vi "test Ntrip-Client.vi"() -> ()   [LabVIEW 2019]
uses:
  <vilib>/Instr/_visa.llb/VISA Configure Serial Port (Instr).vi
panel:
  in  "탭 컨트롤":enum32{"Main", "ref"}(tab)
  out "RTCM recv":string
  in  "address":string="gnss.eseoul.go.kr"
  in  "remote port":u16=2101
  in  "bytes to read":i32=100000
  in  "stop":bool
  in  "VISA resource name":refnum<visa-resource-name> caption="GNSS port"
  in  "정지":bool
  in  "baud rate (9600)":u32=9600 caption="rate"
  in  "불리언":bool
  in  "데이터 입력":string
  # "GET /YONS-RTCM32-M5 HTTP/1.0\nUser-Agent: NTRIP YbbaekRLmodelNTRIPClient/20210615\nAccept: */*\nConnection: close\n\nAuthorization: Basic c2VvdWw6c2VvdWw="
  # "4745 5420 2F59 4F4E 532D 5254 434D 3332 2D4D 3520 4854 5450 2F31 2E30 0D0A 5573 6572 2D41 6765 6E74 3A20 4E54 5249 5020 4C65 6665 6275 7265 4E54 5249 5043 6C69 656E 742F 3230 3133 3131 3234 0D0A 4163 6365 7074 3A20 2A2F 2A0D 0A43 6F6E 6E65 6374 696F 6E3A 2063 6C6F 7365 0A0D 4175 7468 6F72 697A 6174 696F 6E3A 2042 6173 6963 2063 3256 7664 5777 3663 3256 7664 5777 3D0D 0A0D 0A"
  # "4745 5420 2F59 4F4E 532D 5254 434D 3332 2D4D 3520 4854 5450 2F31 2E30 0D0A 5573 6572 2D41 6765 6E74 3A20 4E54 5249 5020 5962 6261 656B 524C 6D6F 6465 6C4E 5452 4950 436C 6965 6E74 2F32 3031 3331 3132 340D 0A41 6363 6570 743A 202A 2F2A 0D0A 436F 6E6E 6563 7469 6F6E 3A20 636C 6F73 650A 0D41 7574 686F 7269 7A61 7469 6F6E 3A20 4261 7369 6320 6332 5676 6457 7736 6332 5676 6457 773D 0D0A 0D0A"
  # "GET /YONS-RTCM32-M5 HTTP/1.0\nUser-Agent: NTRIP YbbaekRLmodelNTRIPClient/20131124\nAccept: */*\nConnection: close\n\nAuthorization: Basic c2VvdWw6c2VvdWw="
  # "Test Ntrip Client"
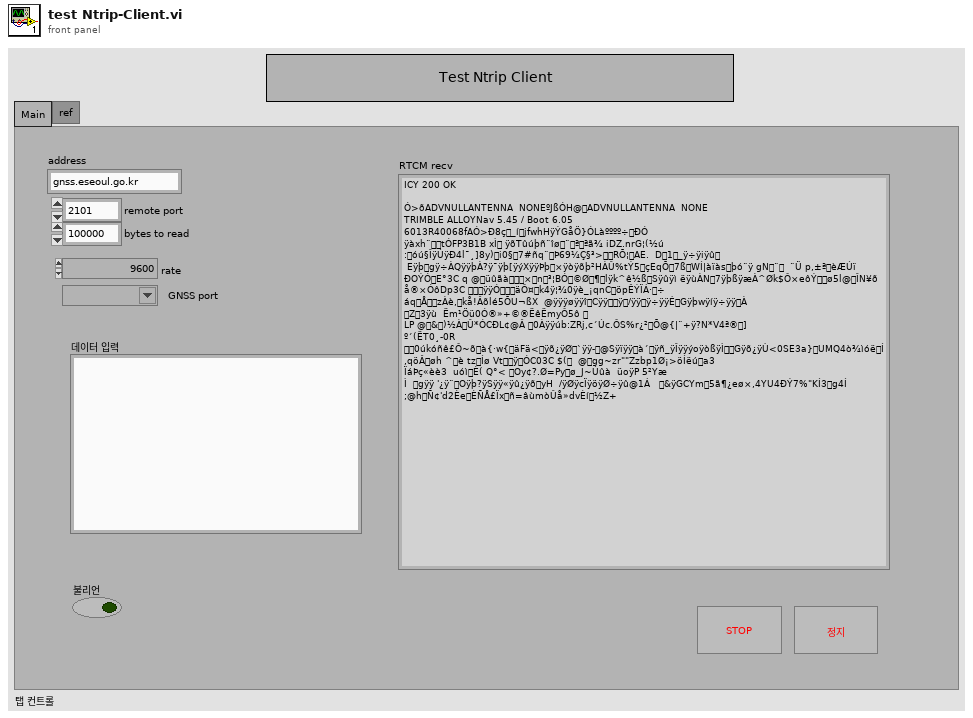
[diagram p1: front panel]
types:
  T1 = enum16{"Standard", "Buffered", "CRLF", "Immediate"}
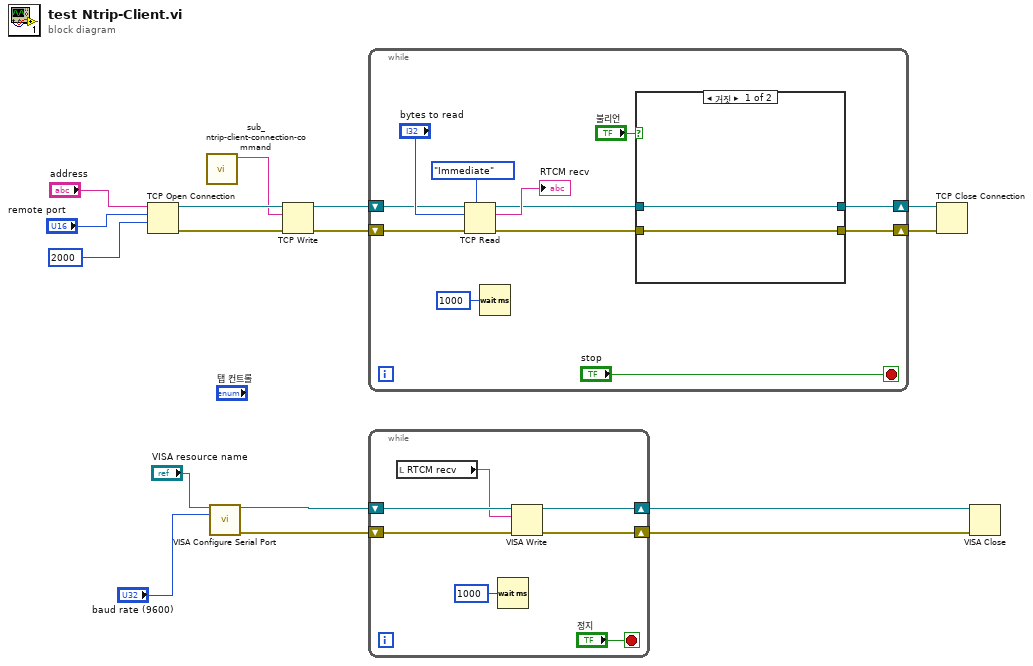
[diagram p0: block diagram]
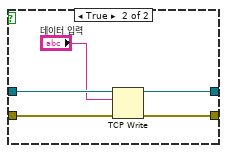
[diagram p2: hidden frame]
diagram:
  n1 = TCP Open Connection(address="address", remote port or service name="remote port", timeout ms (60000)=2000) -> (connection ID=w11:refnum<k5>, error out=w8:errorcluster)  [unwired: 2 in]
  n2 = call "sub_ntrip-client-connection-command.vi"() -> ("String"=w1:string)  [unwired: 11 in]
  n3 = call-poly "VISA Configure Serial Port"("VISA resource name"="VISA resource name", "baud rate (9600)"="baud rate (9600)") -> ("VISA resource name out"=w7:refnum<visa-resource-name>, "error out"=w5:errorcluster)  [unwired: 12 in]
  n4 = TCP Write(connection ID=w11, data in=w1, error in (no error)=w8) -> (connection ID out=w9:refnum<k5>, error out=w10:errorcluster)  [unwired: 1 in, 1 out]
  n5 = while {
    shift-right: [w19] -> w12
    shift-left: w10 -> [w25]
    shift-right: [w18] -> w13
    shift-left: w9 -> [w24]
    stop <- "stop" stop-if-true
    n6 = TCP Read(connection ID=w24, bytes to read="bytes to read", error in (no error)=w25, 7:T1."Immediate" ("mode (standard)")) -> (connection ID out=w20:refnum<k5>, data out=→"RTCM recv":string, error out=w21:errorcluster)  [unwired: 1 in]
    n7 = Wait (ms)(milliseconds to wait=u32 1000) -> ()  [unwired: 1 out]
    n8 = case shown="거짓" "불리언" {
      tunnel: w21 -> [w29 w35]
      tunnel: w20 -> [w30 w34]
      tunnel: [w29 w33] -> w19
      tunnel: [w30 w32] -> w18
      frame False {
      }
      frame True {
        n9 = TCP Write(connection ID=w34, data in="데이터 입력", error in (no error)=w35) -> (connection ID out=w32:refnum<k5>, error out=w33:errorcluster)  [unwired: 1 in, 1 out]
      }
    }
  }
  n10 = while {
    shift-right: [w41] -> w6
    shift-left: w7 -> [w42]
    shift-right: [w39] -> w4
    shift-left: w5 -> [w40]
    stop <- "정지" stop-if-true
    n11 = local read "RTCM recv"() -> (w36:string)
    n12 = Wait (ms)(milliseconds to wait=u32 1000) -> ()  [unwired: 1 out]
    n13 = VISA Write(VISA resource name=w42, write buffer=w36, error in (no error)=w40) -> (VISA resource name out=w41:refnum<visa-resource-name>, error out=w39:errorcluster)  [unwired: 1 out]
  }
  n14 = TCP Close Connection(connection ID=w13, error in (no error)=w12) -> ()  [unwired: 1 in, 2 out]
  n15 = VISA Close(VISA resource name=w6, error in (no error)=w4) -> ()  [unwired: 1 out]
